vi "自动发送实时数据.vi"() -> ()   [LabVIEW 2016]
panel:
  out "error IO":errorcluster
  in  "最低水平":dbl=0.1 format="%#_13g"
  in  "本地端口(0)":u16
  in  "停止按钮":bool
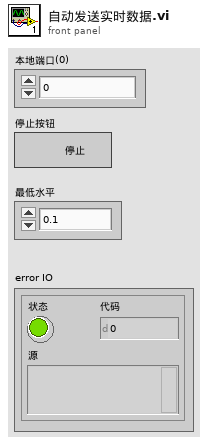
[diagram p1: front panel]
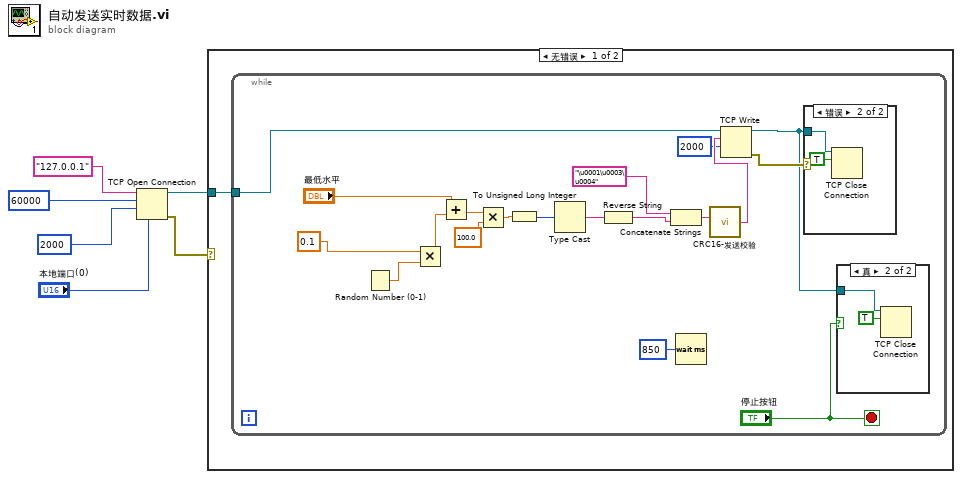
[diagram p0: block diagram]
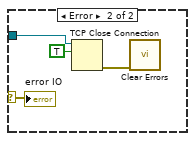
[diagram p4: hidden frame]
diagram:
  n1 = TCP Open Connection(address="127.0.0.1" ("地址"), remote port or service name=u16 60000 ("远程端口或服务名称"), timeout ms (60000)=2000 ("超时毫秒(60000)"), local port="本地端口(0)") -> (connection ID=w3:refnum<k5>, error out=w2:errorcluster)  [unwired: 1 in]
  n2 = case shown="无错误" w2 {
    selector: w2 -> [_ w31]
    tunnel: w3 -> [w7 w33]
    frame No Error {
      n3 = while {
        tunnel: w7 -> [w14]
        stop <- "停止按钮" stop-if-true
        n4 = Random Number (0-1)() -> (number: 0 to 1=w26:dbl)
        n5 = Multiply(x=0.1, y=w26) -> (x*y=w23:dbl)
        n6 = Add(x="最低水平", y=w23) -> (x+y=w22:dbl)
        n7 = Multiply(x=w22, y=100.0) -> (x*y=w20:dbl)
        n8 = To Unsigned Long Integer(number=w20) -> (unsigned 32bit integer=w19:u32)
        n9 = Type Cast(x=w19) -> (*(type *) &x=w18:string)  [unwired: 1 in]
        n10 = Reverse String(1:w18) -> (0:w17:string)
        n11 = Concatenate Strings("\u0001\u0003\u0004" ("字符串"), w17) -> (w15:string)
        n12 = Wait (ms)(milliseconds to wait=u32 850 ("等待时间（毫秒）")) -> ()  [unwired: 1 out]
        n13 = call "CRC16-发送校验.vi"("净数据"=w15) -> ("完整输出"=w12:string)
        n14 = TCP Write(connection ID=w14, data in=w12, 9:2000 ("超时毫秒(25000)")) -> (connection ID out=w9:refnum<k5>, error out=w10:errorcluster)  [unwired: 1 in, 1 out]
        n15 = case shown="错误" w10 {
          tunnel: w9 -> [_ w30]
          frame No Error {
          }
          frame Error {
            n16 = TCP Close Connection(connection ID=w30, abort (F)=TRUE ("中止(F)")) -> ()  [unwired: 1 in, 2 out]
          }
        }
        n17 = case shown="真" "停止按钮" {
          tunnel: w9 -> [_ w28]
          frame False {
          }
          frame True {
            n18 = TCP Close Connection(connection ID=w28, abort (F)=TRUE ("中止(F)")) -> ()  [unwired: 1 in, 2 out]
          }
        }
      }
    }
    frame Error {
      n19 = TCP Close Connection(connection ID=w33, abort (F)=TRUE ("中止(F)")) -> (error out=w32:errorcluster)  [unwired: 1 in, 1 out]
      n20 = call <vilib>:"Clear Errors.vi"("error in (no error)"=w32) -> ()  [unwired: 5 in, 2 out]
      "error IO" <- w31
    }
  }
